vi "Platform System Date.vi"(8 "error in (no error)":errorcluster, 10 "System Date (2010/01/01)":timestamp=timestamp(3345148800 s since 1904-01-01) format="%<%Y/%m/%d>T", 11 "VISA resource name":refnum<visa-resource-name>) -> (0 "error out":errorcluster, 3 "VISA resource name out":refnum<visa-resource-name>)   [LabVIEW 2018, in "LTB-1.lvlib" / "3150.lvlib"]
doc: "Sets the device's internal calendar."
uses:
  3150.lvlib
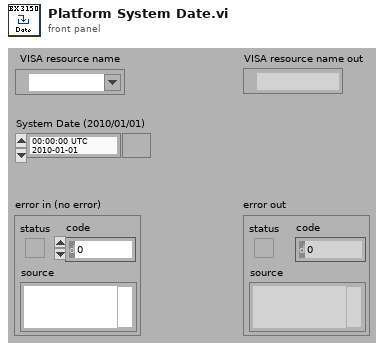
[diagram p1: front panel]
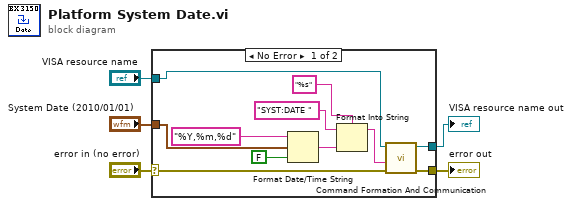
[diagram p0: block diagram]
diagram:
  n1 = case shown="No Error" "error in (no error)" {
    selector: "error in (no error)" -> [w16 w18]
    tunnel: [w15 w18] -> w3
    tunnel: "VISA resource name" -> [w14 w17]
    tunnel: [w13 w17] -> w4
    tunnel: "System Date (2010/01/01)" -> [w8 _]
    frame No Error {
      n2 = Format Date/Time String(time format string (%c)="%Y,%m,%d", seconds (now)=w8, UTC format=FALSE) -> (date/time string=w6:string)
      n3 = Format Into String(format string="%s", initial string="SYST:DATE " ("Command"), w6) -> (resulting string=w11:string)  [unwired: 1 in, 1 out]
      n4 = call "Command Formation And Communication.vi"("error in (no error)"=w16, "Command"=w11, "VISA resource name"=w14) -> ("error out"=w15:errorcluster, "VISA resource name out"=w13:refnum<visa-resource-name>)  [unwired: 1 in, 6 out]
    }
    frame Error {
    }
  }
  "VISA resource name out" <- w4
  "error out" <- w3
